vi "taper_pulling.vi"(0 "VISAsession":refnum<visa-resource-name>="USB0::0x2184::0x0008::3114106::INSTR", 1 "Initialize?":bool=TRUE, 2 "Close?":bool=TRUE, 5 "Output(ON)":bool=TRUE, 7 "Output Set":T3={"Select Mode"=0, "Select Range(100V)"=enum."100V", "Frequency[Hz]"=50.0, "Initial Voltage[Vpp]/[Vrms]"=0.0, "Offset[V]"=0.0} {"Offset[V]" min=-440.0 max=440.0 step=0.1 format="%.1f"; "Initial Voltage[Vpp]/[Vrms]" min=0.0 max=880.0 step=0.1 format="%.1f"; "Frequency[Hz]" min=1.0 max=550.0 step=0.1 format="%.1f"; "Select Mode" items=["AC-INT", "AC-EXT", "AC-ADD", "AC-SYNC", "ACDC-INT", "ACDC-EXT", "ACDC-ADD", "ACDC-SYNC"]}, 9 "Function Set":cluster{"Select Function":u32} {"Select Function" items=["SIN", "SQU", "ARB1", "ARB2", "ARB3", "ARB4", "ARB5", "ARB6", "ARB7", "ARB8", "ARB9", "ARB10", "ARB11", "ARB12", "ARB13", "ARB14", "ARB15", "ARB16"]}, 11 "error in (no error)":errorcluster, 12 "Limit Set":T2={"Limit?"=TRUE, "Average[A]"=6.2, "High[A]"=15.0, "Low[A]"=-15.0} {"Low[A]" min=-42.0 max=-5.0 step=0.1 format="%.1g"; "High[A]" min=5.0 max=42.0 step=0.1 format="%.1g"; "Average[A]" min=1.0 max=10.5 step=0.1 format="%.1g"}) -> (4 "CopyVISAsession":refnum<visa-resource-name>, 6 "ID":string, 8 "Measure":T1, 15 "error out":errorcluster)   [LabVIEW 2019]
doc: "Make the basic output setting, then turn on the output.\nAfter that, use the measurement function to read the measured output value.\n\nNote:\nVoltage Range\nAPS-1102 : 0.0 - 140.0 ( 0.0 - 280.0 ) [Vrms] / 0.0 - 400.0 ( 0.0 - 800.0 ) [Vpp]\nAPS-1102A : 0.0 - 155.0 ( 0.0 - 310.0 ) [Vrms] / 0.0 - 440.0 ( 0.0 - 880.0 ) [Vpp]\n\nOffset Range\nAPS-1102 : -200.0 - +200.0 ( -400.0 - +400.0 ) [V]\nAPS-1102A : -220.0 - +220.0 ( -440.0 - +440.0 ) [V] \n\nCurrent Limit-High Range\nAPS-1102 : +10.0 - +42.0 ( +5.0 - +21.0 ) [A]\nAPS-1102A : +10.0 - +42.0 ( +5.0 - +21.0 ) [A] \n\nCurrent Limit-Low Range\nAPS-1102: -42.0 - -10.0 ( -21.0 - -5.0 ) [A]\nAPS-1102A : -42.0 - -10.0 ( -21.0 - -5.0 ) [A]"
uses:
  <vilib>/Instr/_visa.llb/VISA Configure Serial Port (Instr).vi
panel:
  out "Status":string
  out "error (Puller)":errorcluster
  in  "heater back speed":string="0.2"
  in  "Pulling Motor":string="-14.75,-14.75"
  in  "Pulling speed":string="0.2"
  in  "Heater Position":string="-22"
  in  "High Voltage (V)":i32=16
  # "GettingStarted"
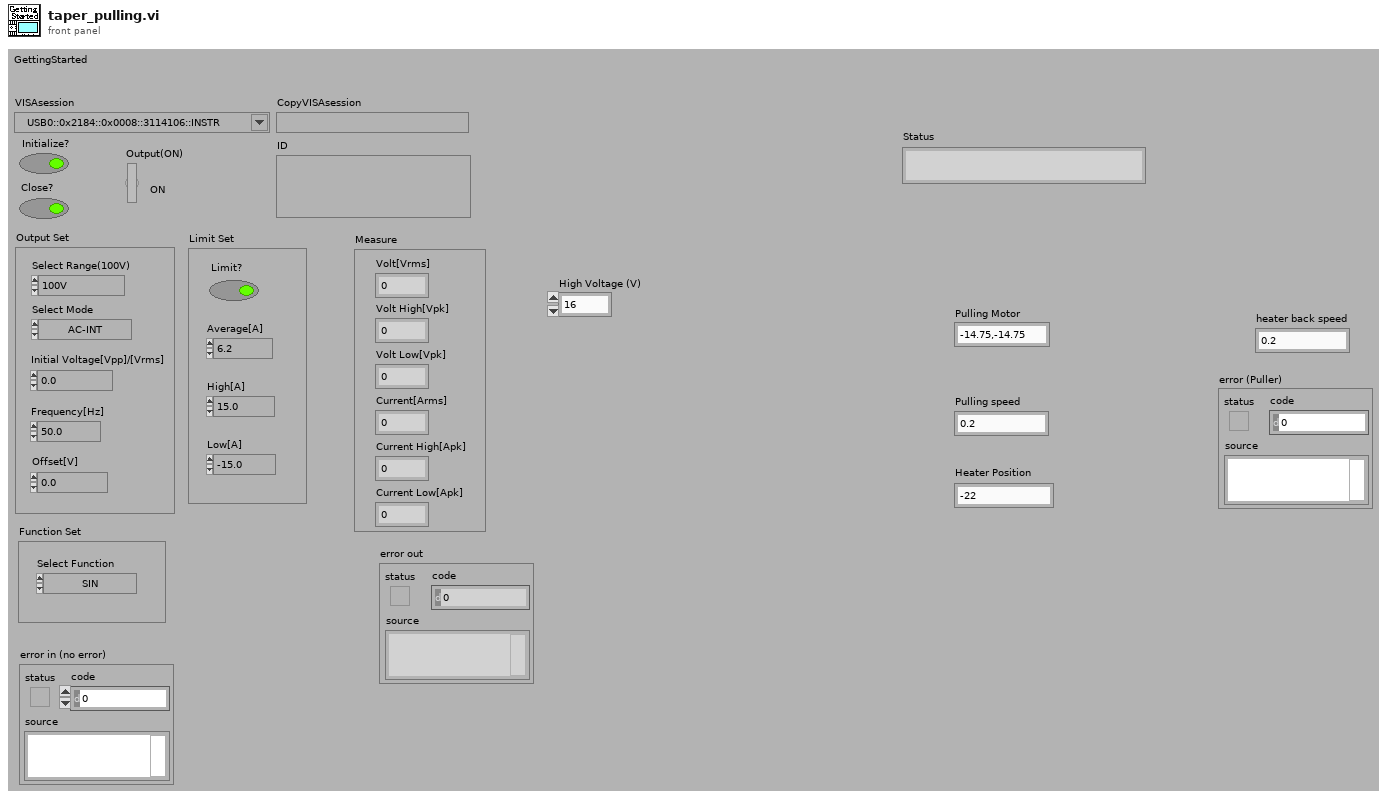
[diagram p1: front panel]
types:
  T1 = cluster{"Volt[Vrms]":dbl, "Volt High[Vpk]":i32, "Volt Low[Vpk]":i32, "Current[Arms]":dbl, "Current High[Apk]":dbl, "Current Low[Apk]":dbl}
  T2 = cluster{"Limit?":bool, "Average[A]":dbl, "High[A]":dbl, "Low[A]":dbl}
  T3 = cluster{"Select Mode":u32, "Select Range(100V)":enum16{"100V", "200V"}, "Frequency[Hz]":dbl, "Initial Voltage[Vpp]/[Vrms]":dbl, "Offset[V]":dbl}
  T4 = cluster{"Voltage:AC+DC":dbl, "Peak High:AC+DC":i32, "Peak Low:AC+DC":i32, "Current:AC+DC":dbl, "Peak High:AC+DC":dbl, "Peak Low:AC+DC":dbl}
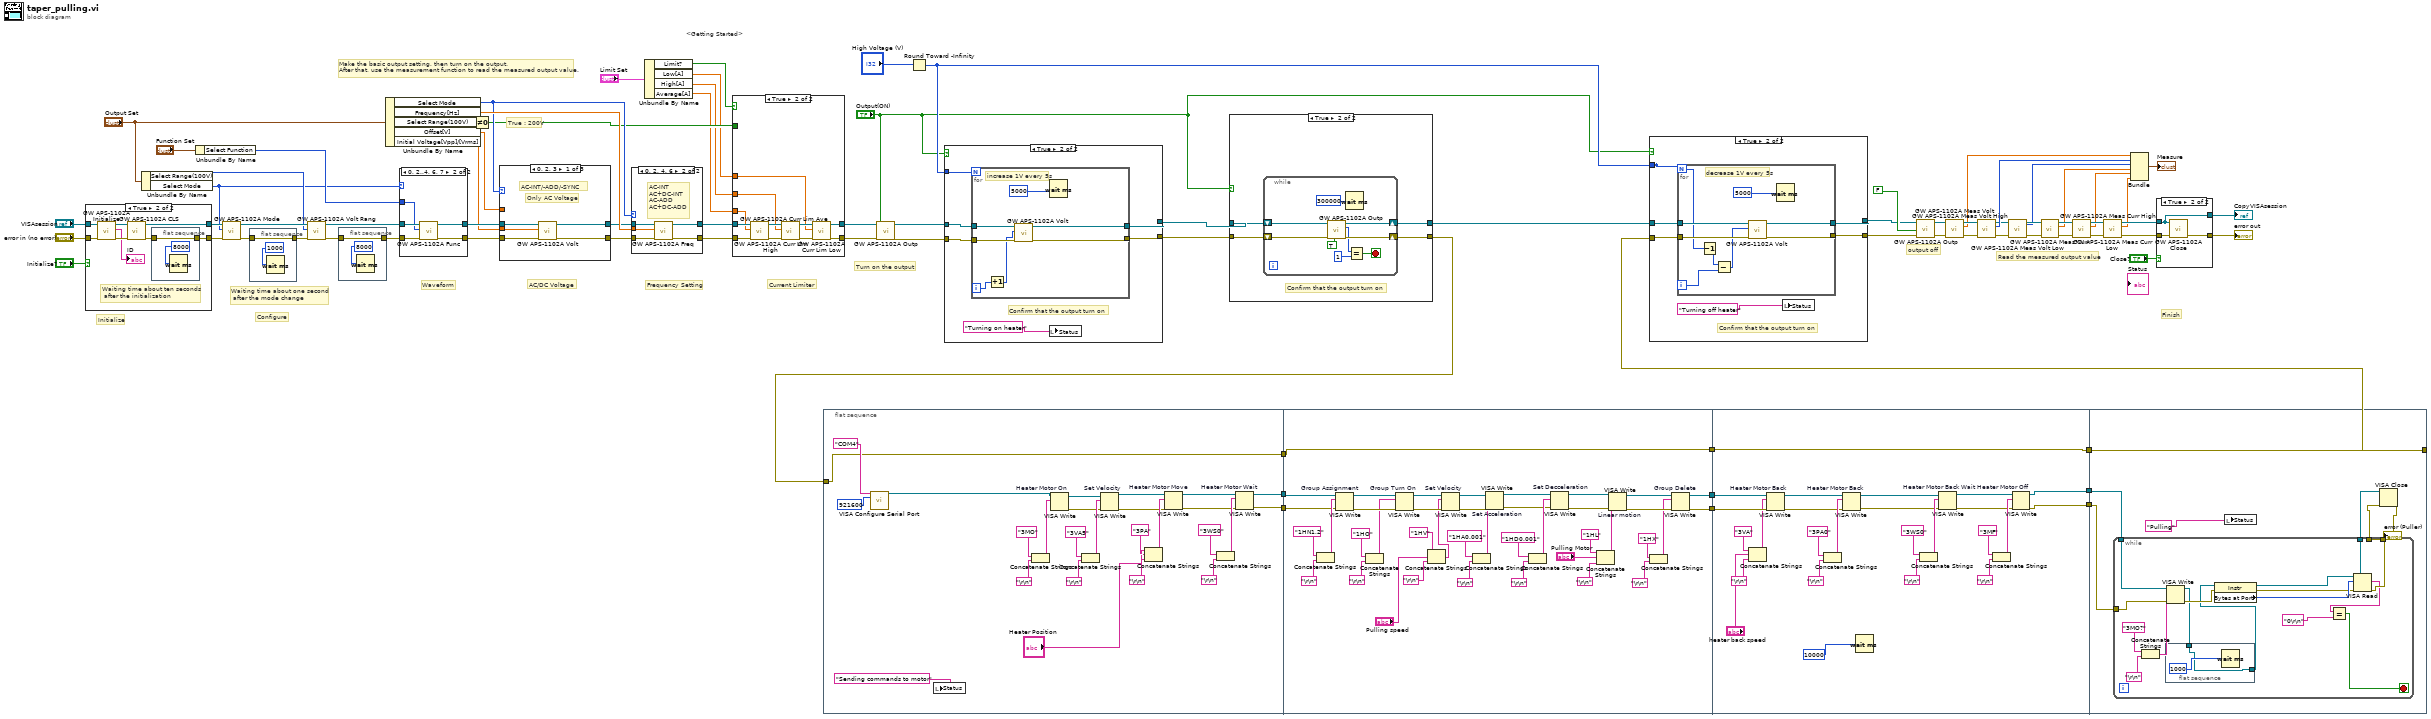
[diagram p0: block diagram]
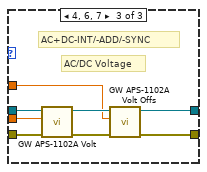
[diagram p6: hidden frame]
diagram:
  # "output off"
  # "Waiting time about one second\n after the mode change"
  # "True : 200V"
  # "Frequency Setting"
  # "<Getting Started>"
  # "Finish"
  # "Make the basic output setting, then turn on the output.\nAfter that, use the measurement function to read the measured output value."
  # "Turn on the output"
  # "Read the measured output value"
  # "Current Limiter"
  # "Waveform"
  # "AC/DC Voltage"
  # "Configure"
  # "Initialize"
  n1 = case shown="True" "Initialize?" {
    tunnel: "VISAsession" -> [w83 w91]
    tunnel: [w83 w88] -> w69
    tunnel: [w82 w85] -> w70
    tunnel: "error in (no error)" -> [w82 w86]
    frame False {
    }
    frame True {
      # "Waiting time about ten seconds\n after the initialization"
      n2 = call "GW APS-1102A Initialize.vi"("error in (no error)"=w86, "VISAsession"=w91) -> ("error out"=w89:errorcluster, "ID"=→"ID":string, "CopyVISAsession"=w90:refnum<visa-resource-name>)  [unwired: 7 in]
      n3 = call "GW APS-1102A CLS.vi"("error in (no error)"=w89, "VISAsession"=w90) -> ("error out"=w84:errorcluster, "CopyVISAsession"=w88:refnum<visa-resource-name>)  [unwired: 8 in]
      n4 = flat-sequence {
        tunnel: w84 -> [w92]
        tunnel: [w92] -> w85
        frame #0 {
          n5 = Wait (ms)(milliseconds to wait=u32 8000) -> ()  [unwired: 1 out]
        }
      }
    }
  }
  n6 = Unbundle By Name("Output Set") -> ("Select Range(100V)"=w67:enum16{"100V", "200V"}, "Select Mode"=w54:u32)
  n7 = Unbundle By Name("Function Set") -> ("Select Function"=w55:u32)
  n8 = call "GW APS-1102A Mode.vi"("error in (no error)"=w70, "Select Mode"=w54, "VISAsession"=w69) -> ("error out"=w31:errorcluster, "CopyVISAsession"=w68:refnum<visa-resource-name>)  [unwired: 6 in, 1 out]
  n9 = flat-sequence {
    tunnel: [w94] -> w30
    tunnel: w31 -> [w94]
    frame #0 {
      n10 = Wait (ms)(milliseconds to wait=u32 1000) -> ()  [unwired: 1 out]
    }
  }
  n11 = call "GW APS-1102A Volt Rang.vi"("error in (no error)"=w30, "Select Range(100V)"=w67, "VISAsession"=w68) -> ("error out"=w27:errorcluster, "CopyVISAsession"=w56:refnum<visa-resource-name>)  [unwired: 6 in, 1 out]
  n12 = flat-sequence {
    tunnel: w27 -> [w96]
    tunnel: [w96] -> w26
    frame #0 {
      n13 = Wait (ms)(milliseconds to wait=u32 8000) -> ()  [unwired: 1 out]
    }
  }
  n14 = Unbundle By Name("Output Set") -> ("Select Mode"=w61:u32, "Frequency[Hz]"=w66:dbl, "Select Range(100V)"=w53:enum16{"100V", "200V"}, "Offset[V]"=w59:dbl, "Initial Voltage[Vpp]/[Vrms]"=w60:dbl)
  n15 = case shown="0, 2..4, 6, 7" w54 {
    tunnel: w56 -> [w99 w103]
    tunnel: w26 -> [w98 w104]
    tunnel: [w99 w101] -> w65
    tunnel: [w98 w100] -> w64
    tunnel: w55 -> [_ w102]
    frame 1, 5, Default {
      # "AC-EXT\nAC+DC-EXT"
    }
    frame 0, 2..4, 6, 7 {
      n16 = call "GW APS-1102A Func.vi"("error in (no error)"=w104, "Select Function"=w102, "VISAsession"=w103) -> ("error out"=w100:errorcluster, "CopyVISAsession"=w101:refnum<visa-resource-name>)  [unwired: 6 in, 1 out]
    }
  }
  n17 = Not Equal To 0?(x=w53) -> (x != 0?=w52:bool)
  n18 = case shown="0, 2, 3" w61 {
    tunnel: w65 -> [w107 w111 w114]
    tunnel: w64 -> [w106 w110 w115]
    tunnel: [w109 w111 w119] -> w63
    tunnel: [w108 w110 w118] -> w62
    tunnel: w60 -> [w105 _ w113]
    tunnel: w59 -> [_ _ w112]
    frame 0, 2, 3 {
      # "Only AC Voltage"
      # "AC-INT/-ADD/-SYNC"
      n19 = call "GW APS-1102A Volt.vi"("error in (no error)"=w106, "Voltage[Vpp]/[Vrms]"=w105, "VISAsession"=w107) -> ("error out"=w108:errorcluster, "CopyVISAsession"=w109:refnum<visa-resource-name>)  [unwired: 5 in, 2 out]
    }
    frame 1, 5, Default {
      # "AC-EXT\nAC+DC-EXT"
    }
    frame 4, 6, 7 {
      # "AC/DC Voltage"
      # "AC+DC-INT/-ADD/-SYNC"
      n20 = call "GW APS-1102A Volt.vi"("error in (no error)"=w115, "Voltage[Vpp]/[Vrms]"=w113, "VISAsession"=w114) -> ("error out"=w117:errorcluster, "CopyVISAsession"=w116:refnum<visa-resource-name>)  [unwired: 5 in, 2 out]
      n21 = call "GW APS-1102A Volt Offs.vi"("error in (no error)"=w117, "Offset(0)"=w112, "VISAsession"=w116) -> ("error out"=w118:errorcluster, "CopyVISAsession"=w119:refnum<visa-resource-name>)  [unwired: 5 in, 2 out]
    }
  }
  n22 = case shown="0, 2, 4, 6" w61 {
    tunnel: [w121 w126] -> w58
    tunnel: [w120 w125] -> w57
    tunnel: w62 -> [w120 w124]
    tunnel: w63 -> [w121 w123]
    tunnel: w66 -> [_ w122]
    frame 1, 3, 5, 7, Default {
      # "AC-EXT\nAC+DC-EXT\nAC-SYNC\nAC+DC-SYNC"
    }
    frame 0, 2, 4, 6 {
      # "AC-INT\nAC+DC-INT\nAC-ADD\nAC+DC-ADD"
      n23 = call "GW APS-1102A Freq.vi"("error in (no error)"=w124, "Frequency(1)"=w122, "VISAsession"=w123) -> ("error out"=w125:errorcluster, "CopyVISAsession"=w126:refnum<visa-resource-name>)  [unwired: 5 in, 2 out]
    }
  }
  n24 = Unbundle By Name("Limit Set") -> ("Limit?"=w71:bool, "Low[A]"=w49:dbl, "High[A]"=w50:dbl, "Average[A]"=w51:dbl)
  n25 = case shown="True" w71 {
    tunnel: [w128 w132] -> w80
    tunnel: [w127 w134] -> w78
    tunnel: w58 -> [w128 w137]
    tunnel: w57 -> [w127 w136]
    tunnel: w52 -> [_ _]
    tunnel: w51 -> [_ w131]
    tunnel: w50 -> [_ w130]
    tunnel: w49 -> [_ w129]
    frame False {
    }
    frame True {
      n26 = call "GW APS-1102A Curr Lim Ave.vi"("error in (no error)"=w136, "Average(5.3)"=w131, "VISAsession"=w137) -> ("error out"=w138:errorcluster, "CopyVISAsession"=w139:refnum<visa-resource-name>)  [unwired: 5 in, 2 out]
      n27 = call "GW APS-1102A Curr Lim High.vi"("error in (no error)"=w138, "High(21)"=w130, "VISAsession"=w139) -> ("error out"=w135:errorcluster, "CopyVISAsession"=w133:refnum<visa-resource-name>)  [unwired: 5 in, 2 out]
      n28 = call "GW APS-1102A Curr Lim Low.vi"("error in (no error)"=w135, "Low(-21)"=w129, "VISAsession"=w133) -> ("error out"=w134:errorcluster, "CopyVISAsession"=w132:refnum<visa-resource-name>)  [unwired: 5 in, 2 out]
    }
  }
  n29 = flat-sequence {
    tunnel: [w147] -> w11
    tunnel: [w146] -> w10
    tunnel: w7 -> [w142]
    tunnel: [w142] -> w4
    tunnel: w11 -> [w179]
    tunnel: [w173] -> w9
    tunnel: [w175] -> w8
    tunnel: w10 -> [w171]
    tunnel: [w166] -> w5
    tunnel: w4 -> [w166]
    tunnel: w9 -> [w218]
    tunnel: w8 -> [w219]
    tunnel: w5 -> [w209]
    tunnel: [w209] -> w3
    tunnel: [w208] -> w2
    tunnel: [w207] -> w1
    tunnel: [w237] -> w6
    tunnel: w3 -> [w237]
    tunnel: w2 -> [w235]
    tunnel: w1 -> [w234]
    frame #0 {
      n30 = call-poly "VISA Configure Serial Port"("VISA resource name"="COM4" ("string"), "baud rate (9600)"=u32 921600) -> ("VISA resource name out"=w141:refnum<visa-resource-name>)  [unwired: 12 in, 1 out]
      n31 = local write "Status"("Sending commands to motor" ("string")) -> ()
      n32 = Concatenate Strings("3MO" ("string"), "\r\n") -> (w162:string)
      n33 = VISA Write "Heater Motor On"(VISA resource name=w141, write buffer=w162) -> (VISA resource name out=w158:refnum<visa-resource-name>, error out=w155:errorcluster)  [unwired: 1 in, 1 out]
      n34 = Concatenate Strings("3VA5" ("string"), "\r\n") -> (w159:string)
      n35 = VISA Write "Set Velocity"(VISA resource name=w158, write buffer=w159, error in (no error)=w155) -> (VISA resource name out=w154:refnum<visa-resource-name>, error out=w153:errorcluster)  [unwired: 1 out]
      n36 = Concatenate Strings("3PA" ("string"), "Heater Position", "\r\n") -> (w157:string)
      n37 = VISA Write "Heater Motor Move"(VISA resource name=w154, write buffer=w157, error in (no error)=w153) -> (VISA resource name out=w149:refnum<visa-resource-name>, error out=w148:errorcluster)  [unwired: 1 out]
      n38 = Concatenate Strings("3WS0" ("string"), "\r\n") -> (w152:string)
      n39 = VISA Write "Heater Motor Wait"(VISA resource name=w149, write buffer=w152, error in (no error)=w148) -> (VISA resource name out=w147:refnum<visa-resource-name>, error out=w146:errorcluster)  [unwired: 1 out]
    }
    frame #1 {
      n40 = Concatenate Strings("1HN1,2" ("string"), "\r\n") -> (w204:string)
      n41 = VISA Write "Group Assignment"(VISA resource name=w179, write buffer=w204, error in (no error)=w171) -> (VISA resource name out=w201:refnum<visa-resource-name>, error out=w205:errorcluster)  [unwired: 1 out]
      n42 = Concatenate Strings("1HO" ("string"), "\r\n") -> (w182:string)
      n43 = VISA Write "Group Turn On"(VISA resource name=w201, write buffer=w182, error in (no error)=w205) -> (VISA resource name out=w187:refnum<visa-resource-name>, error out=w188:errorcluster)  [unwired: 1 out]
      n44 = Concatenate Strings("1HV" ("string"), "Pulling speed", "\r\n") -> (w170:string)
      n45 = VISA Write "Set Velocity"(VISA resource name=w187, write buffer=w170, error in (no error)=w188) -> (VISA resource name out=w192:refnum<visa-resource-name>, error out=w193:errorcluster)  [unwired: 1 out]
      n46 = Concatenate Strings("1HA0.001" ("string"), "\r\n") -> (w191:string)
      n47 = VISA Write "Set Acceleration"(VISA resource name=w192, write buffer=w191, error in (no error)=w193) -> (VISA resource name out=w197:refnum<visa-resource-name>, error out=w195:errorcluster)  [unwired: 1 out]
      n48 = Concatenate Strings("1HD0.001" ("string"), "\r\n") -> (w198:string)
      n49 = VISA Write "Set Decceleration"(VISA resource name=w197, write buffer=w198, error in (no error)=w195) -> (VISA resource name out=w186:refnum<visa-resource-name>, error out=w185:errorcluster)  [unwired: 1 out]
      n50 = Concatenate Strings("1HL" ("string"), "Pulling Motor", "\r\n") -> (w184:string)
      n51 = VISA Write "Linear motion"(VISA resource name=w186, write buffer=w184, error in (no error)=w185) -> (VISA resource name out=w174:refnum<visa-resource-name>, error out=w176:errorcluster)  [unwired: 1 out]
      n52 = Concatenate Strings("1HX" ("string"), "\r\n") -> (w172:string)
      n53 = VISA Write "Group Delete"(VISA resource name=w174, write buffer=w172, error in (no error)=w176) -> (VISA resource name out=w173:refnum<visa-resource-name>, error out=w175:errorcluster)  [unwired: 1 out]
    }
    frame #2 {
      n54 = Concatenate Strings("3VA" ("string"), "heater back speed", "\r\n") -> (w213:string)
      n55 = VISA Write "Heater Motor Back"(VISA resource name=w218, write buffer=w213, error in (no error)=w219) -> (VISA resource name out=w217:refnum<visa-resource-name>, error out=w216:errorcluster)  [unwired: 1 out]
      n56 = Concatenate Strings("3PA0" ("string"), "\r\n") -> (w230:string)
      n57 = VISA Write "Heater Motor Back"(VISA resource name=w217, write buffer=w230, error in (no error)=w216) -> (VISA resource name out=w215:refnum<visa-resource-name>, error out=w214:errorcluster)  [unwired: 1 out]
      n58 = Wait (ms)(milliseconds to wait=10000) -> ()  [unwired: 1 out]
      n59 = Concatenate Strings("3WS0" ("string"), "\r\n") -> (w224:string)
      n60 = VISA Write "Heater Motor Back Wait"(VISA resource name=w215, write buffer=w224, error in (no error)=w214) -> (VISA resource name out=w221:refnum<visa-resource-name>, error out=w220:errorcluster)  [unwired: 1 out]
      n61 = Concatenate Strings("3MF" ("string"), "\r\n") -> (w227:string)
      n62 = VISA Write "Heater Motor Off"(VISA resource name=w221, write buffer=w227, error in (no error)=w220) -> (VISA resource name out=w207:refnum<visa-resource-name>, error out=w208:errorcluster)  [unwired: 1 out]
    }
    frame #3 {
      n63 = while {
        tunnel: w235 -> [w252]
        tunnel: w234 -> [w249]
        tunnel: [w246] -> w233
        tunnel: [w247] -> w232
        tunnel: [w246] -> _
        stop <- w239 stop-if-true
        n64 = Concatenate Strings("3MO?" ("string"), "\r\n") -> (w243:string)
        n65 = flat-sequence {
          tunnel: w242 -> [w254]
          tunnel: [w254] -> w241
          frame #0 {
            n66 = Wait (ms)(milliseconds to wait=1000) -> ()  [unwired: 1 out]
          }
        }
        n67 = VISA Write(VISA resource name=w249, write buffer=w243, error in (no error)=w252) -> (VISA resource name out=w242:refnum<visa-resource-name>, error out=w251:errorcluster)  [unwired: 1 out]
        n68 = property class="Instr"(reference=w241, error in=w251) -> (reference out=w248:refnum<visa-resource-name>, error out=w250:errorcluster, "Bytes at Port"=w253:u32)
        n69 = VISA Read(VISA resource name=w248, byte count=w253, error in (no error)=w250) -> (VISA resource name out=w247:refnum<visa-resource-name>, read buffer=w238:string, error out=w246:errorcluster)  [unwired: 1 out]
        n70 = Equal?(x=w238, y="0\r\n") -> (x = y?=w239:bool)
      }
      n71 = local write "Status"("Pulling") -> ()
      n72 = VISA Close(VISA resource name=w232, error in (no error)=w233) -> (error out=→"error (Puller)":errorcluster)
    }
  }
  n73 = call "GW APS-1102A Outp.vi"("error in (no error)"=w78, "State(OFF)"="Output(ON)", "VISAsession"=w80) -> ("error out"=w23:errorcluster, "CopyVISAsession"=w21:refnum<visa-resource-name>)  [unwired: 5 in, 2 out]
  n74 = Round Toward -Infinity(1:"High Voltage (V)") -> (0:w18:i32)
  n75 = case shown="True" "Output(ON)" {
    tunnel: w18 -> [_ w263]
    tunnel: [w256 w259] -> w20
    tunnel: w23 -> [w257 w262]
    tunnel: [w257 w261] -> w22
    tunnel: w21 -> [w256 w260]
    frame False {
    }
    frame True {
      # "Confirm that the output turn on"
      n76 = for {
        N: w263 -> [_]
        tunnel: w262 -> [w270]
        tunnel: [w267] -> w261
        tunnel: w260 -> [w269]
        tunnel: [w268] -> w259
        i -> [w265]
        # "increase 1V every 5s"
        n77 = Increment(x=w265) -> (x+1=w264:i32)
        n78 = call "GW APS-1102A Volt.vi"("error in (no error)"=w270, "Voltage[Vpp]/[Vrms]"=w264, "VISAsession"=w269) -> ("error out"=w267:errorcluster, "CopyVISAsession"=w268:refnum<visa-resource-name>)  [unwired: 5 in, 2 out]
        n79 = Wait (ms)(milliseconds to wait=u32 5000) -> ()  [unwired: 1 out]
      }
      n80 = local write "Status"("Turning on heater") -> ()
    }
  }
  n81 = case shown="True" "Output(ON)" {
    tunnel: w20 -> [w272 w276]
    tunnel: w22 -> [w271 w275]
    tunnel: [w271 w274] -> w7
    tunnel: [w272 w273] -> w19
    frame False {
      # "Output : OFF"
    }
    frame True {
      # "Confirm that the output turn on"
      n82 = while {
        shift-right: [w283] -> w274
        shift-left: w275 -> [w285]
        shift-right: [w277] -> w273
        shift-left: w276 -> [w284]
        stop <- w280 stop-if-true
        n83 = call "GW APS-1102A Outp.vi"("Read(F)"=TRUE, "error in (no error)"=w285, "VISAsession"=w284) -> ("error out"=w283:errorcluster, "Query"=w279:i32, "CopyVISAsession"=w277:refnum<visa-resource-name>)  [unwired: 5 in, 1 out]
        n84 = Wait (ms)(milliseconds to wait=u32 300000) -> ()  [unwired: 1 out]
        n85 = Equal?(x=w279, y=1) -> (x = y?=w280:bool)
      }
    }
  }
  n86 = case shown="True" "Output(ON)" {
    tunnel: [_ w289] -> _
    tunnel: [w286 w290] -> w12
    tunnel: w6 -> [w287 w293]
    tunnel: [w287 w292] -> w15
    tunnel: w19 -> [w286 w291]
    tunnel: w18 -> [_ w289]
    frame False {
    }
    frame True {
      # "Confirm that the output turn on"
      n87 = for {
        N: w289 -> [w295]
        tunnel: w293 -> [w302]
        tunnel: [w299] -> w292
        tunnel: w291 -> [w301]
        tunnel: [w300] -> w290
        i -> [w297]
        # "decrease 1V every 5s"
        n88 = Decrement(x=w295) -> (x-1=w294:i32)
        n89 = Subtract(x=w294, y=w297) -> (x-y=w296:i32)
        n90 = call "GW APS-1102A Volt.vi"("error in (no error)"=w302, "Voltage[Vpp]/[Vrms]"=w296, "VISAsession"=w301) -> ("error out"=w299:errorcluster, "CopyVISAsession"=w300:refnum<visa-resource-name>)  [unwired: 5 in, 2 out]
        n91 = Wait (ms)(milliseconds to wait=u32 5000) -> ()  [unwired: 1 out]
      }
      n92 = local write "Status"("Turning off heater") -> ()
    }
  }
  n93 = call "GW APS-1102A Outp.vi"("error in (no error)"=w15, "State(OFF)"=FALSE, "VISAsession"=w12) -> ("error out"=w14:errorcluster, "CopyVISAsession"=w16:refnum<visa-resource-name>)  [unwired: 5 in, 2 out]
  n94 = call "GW APS-1102A Meas Volt.vi"("error in (no error)"=w14, "VISAsession"=w16) -> ("error out"=w45:errorcluster, "Voltage:AC+DC"=w42:dbl, "CopyVISAsession"=w48:refnum<visa-resource-name>)  [unwired: 5 in, 2 out]
  n95 = call "GW APS-1102A Meas Volt High.vi"("error in (no error)"=w45, "VISAsession"=w48) -> ("error out"=w35:errorcluster, "Peak High:AC+DC"=w41:i32, "CopyVISAsession"=w36:refnum<visa-resource-name>)  [unwired: 5 in, 2 out]
  n96 = call "GW APS-1102A Meas Volt Low.vi"("error in (no error)"=w35, "VISAsession"=w36) -> ("error out"=w37:errorcluster, "Peak Low:AC+DC"=w33:i32, "CopyVISAsession"=w38:refnum<visa-resource-name>)  [unwired: 5 in, 2 out]
  n97 = call "GW APS-1102A Meas Curr.vi"("error in (no error)"=w37, "VISAsession"=w38) -> ("error out"=w44:errorcluster, "Current:AC+DC"=w34:dbl, "CopyVISAsession"=w47:refnum<visa-resource-name>)  [unwired: 5 in, 2 out]
  n98 = call "GW APS-1102A Meas Curr High.vi"("error in (no error)"=w44, "VISAsession"=w47) -> ("error out"=w43:errorcluster, "Peak High:AC+DC"=w40:dbl, "CopyVISAsession"=w46:refnum<visa-resource-name>)  [unwired: 5 in, 2 out]
  n99 = call "GW APS-1102A Meas Curr Low.vi"("error in (no error)"=w43, "VISAsession"=w46) -> ("error out"=w77:errorcluster, "Peak Low:AC+DC"=w39:dbl, "CopyVISAsession"=w79:refnum<visa-resource-name>)  [unwired: 5 in, 2 out]
  n100 = Bundle("Voltage:AC+DC"=w42, "Peak High:AC+DC"=w41, "Peak Low:AC+DC"=w33, "Current:AC+DC"=w34, "Peak High:AC+DC"=w40, "Peak Low:AC+DC"=w39) -> (→"Measure":T4)  [unwired: 1 out]
  n101 = case shown="True" "Close?" {
    tunnel: w79 -> [w303 w305]
    tunnel: w77 -> [w304 w307]
    tunnel: [w304 w306] -> w29
    tunnel: [w303 w305] -> w74
    frame False {
    }
    frame True {
      n102 = call "GW APS-1102A Close.vi"("error in (no error)"=w307, "VISAsession"=w305) -> ("error out"=w306:errorcluster)  [unwired: 9 in]
    }
  }
  "CopyVISAsession" <- w74
  "error out" <- w29
